vi "NanotecSMCPD.get axis status.vi"(0 "i ref in":refnum<vi>, 1 "axis":i32, 3 "ms timeout (10000)":i32=10000, 5 "error in (no error)":errorcluster) -> (14 "i ref out":refnum<vi>, 15 "status":T1=1 items=["motorEnabled"=1, "negativeLimitSwitchActive"=2, "positiveLimitSwitchActive"=4, "limitSwitchesEnabled"=8, "limitSwitchesAreNormallyClosed"=16, "moving"=32, "referenced"=64, "inPosition"=128, "reserved2"=256, "reserved3"=512, "reserved4"=1024, "reserved5"=2048, "error"=4096, "reserved6"=8192, "reserved7"=16384, "reserved8"=32768, "user defined1"=65536, "user defined2"=131072, "user defined3"=262144, "user defined4"=524288, "user defined5"=1048576, "user defined6"=2097152, "user defined7"=4194304, "user defined8"=8388608, "user defined9"=16777216, "user defined10"=33554432, "user defined11"=67108864, "user defined12"=134217728, "user defined13"=268435456, "user defined14"=536870912, "user defined15"=1073741824, "user defined16"=2147483648], 16 "motorOn":bool, 17 "timed out":bool, 19 "error out":errorcluster)   [LabVIEW 2014, in "NanotecSMCPD.lvlib"]
doc: "Gets the 32bit status byte of the specified axis."
uses:
  NanotecSMCPD.lvlib
  CSCore/CSApplicationBaseClasses/MotorBase/MotorBase.statusType.ctl
  CSCore/CSSystem/CoreDefs/CoreDefs.error_type.ctl
  CSCore/CSSystem/CoreDefs/CoreDefs.error_severity.ctl
  CSCore/CSApplicationBaseClasses/MotorBase/MotorBase.directionType.ctl
  CSCore/CSApplicationBaseClasses/MotorBase/MotorBase.serviceType.ctl
  CSlibraries/UtilityLib/UtilityLib.valueStatus.ctl
  CSCore/CSApplicationBaseClasses/DeviceBase/DeviceBase.lvlib
  CSCore/CSSystem/CoreLib/CoreLib.lvlib
  CSCore/CSApplicationBaseClasses/MotorBase/MotorBase.lvlib
  CSlibraries/UtilityLib/UtilityLib.lvlib
  CSinstr.lib/NanotecSMCPD/NanotecSMCPDDriver.lvlib
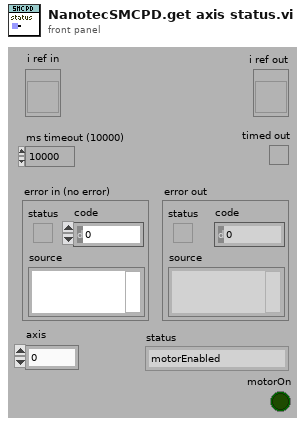
[diagram p1: front panel]
types:
  T1 = typedef "MotorBase.lvlib/MotorBase.statusType.ctl" = u32
  T2 = typedef "CoreDefs.error_severity.ctl" = enum16{"undefined", "information", "warning", "error", "fatal"}
  T3 = typedef "CoreDefs.error_type.ctl" = enum16{"no error", "can't load process", "can't unload process", "process does not exist", "can't install process", "can't remove process", "unknown function", "time out", "can't execute function", "duplicate queue name", "super not found", "caller queue invalid", "can't ping process", "unknown error", "VISA Error", "VISA timeout", "GPIB timeout", "GPIB error", "communication error", "data type mismatch", "can't read data from OPC server", "can't write data to OPC server", "OET error", "function not implemented", "process already exists", "invalid Shared Variable name", "error writing Shared Variable", "error reading Shared Variable", "invalid client name", "corrupt database", "unknown class", "call not authorized", "parameter out of range", "OET timeout: can't get data to modify", "invalid queue name", "requested operation incompatible with current state", "event undefined", "event disabled", "state undefined", "caller is not a friend", "EventBuilder: bad eventID", "EventBuilder: no DAQ devices", "a thread must not stop itself", "UNUSED ELEMENT4", "DiscArchiver: eventData incomplete", "DiscArchiver: eventData does not belong to run", "DiscArchiver: can't open file", "DiscArchiver: can't write to file", "DiscArchiver: available disc space low", "can't acquire semaphore", "error reading data from database", "notifier object is not existing", "can't register process", "can't unregister process", "illegal event type", "object disabled", "object already exists", "can't change state", "Instrument not found", "no connection to remote node", "invalid reference", "N/A", "UNUSED ELEMENT 1", "element not found", "illegal TCP/IP connection detected", "object does not exist", "invalid access ID", "unknown CS system", "invalid privilige", "unsupported data type", "unsupported server type", "IO server already exists", "Shared Variable already exists"}
  T4 = typedef "MotorBase.lvlib/MotorBase.serviceType.ctl" = enum16{"onOff", "startVelocity", "stopVelocity", "acceleration", "rangeMin", "rangeMax", "status", "position"}
  T5 = typedef "UtilityLib.lvlib/UtilityLib.valueStatus.ctl" = enum16{"no info available", "stand by/off", "on", "warning", "alarm/malfunction", "not implemented", "user action required", "important information", "system default", "control default", "indicator default", "button default"}
  T6 = typedef "MotorBase.lvlib/MotorBase.directionType.ctl" = enum16{"unknown", "update actual value", "update nominal value", "update both"}
  T7 = typedef "NanotecSMCPDDriver.lvlib/NanotecSMCPDDriver.status type.ctl" = cluster{"ready":bool, "homePosition":bool, "positionError":bool, "input1":bool, "controllerMode":enum16{"unknown", "position", "speed", "flagPosition", "clockDirection", "analog", "joystick", "unused"}, "unused":bool}
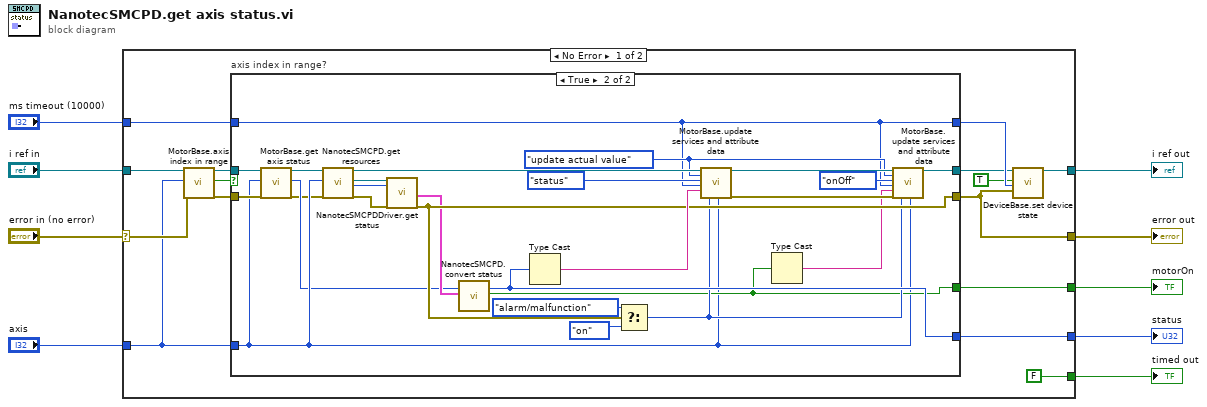
[diagram p0: block diagram]
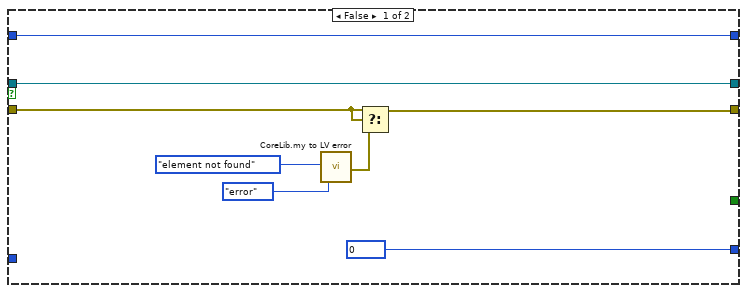
[diagram p2: hidden frame]
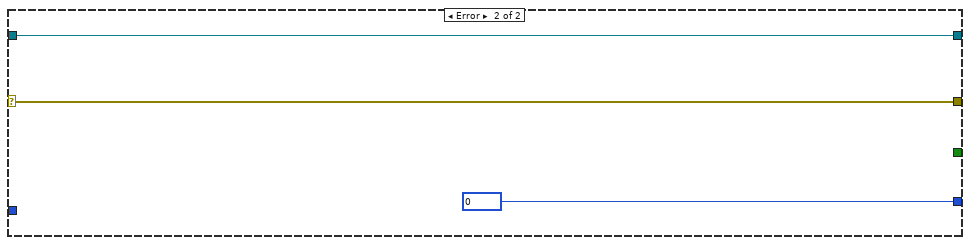
[diagram p3: hidden frame]
diagram:
  n1 = case shown="No Error" "error in (no error)" {
    selector: "error in (no error)" -> [w17 w60]
    tunnel: "ms timeout (10000)" -> [w14 _]
    tunnel: "i ref in" -> [w18 w61]
    tunnel: [w16 w60] -> w6
    tunnel: "axis" -> [w15 _]
    tunnel: [w13 w61] -> w4
    tunnel: [w12 w59] -> w3
    tunnel: [w11 _] -> w2
    tunnel: [FALSE _] -> w1
    frame No Error {
      n2 = call "MotorBase.axis index in range.vi"("i ref in"=w18, "axisIndex"=w15, "error in (no error)"=w17) -> ("i ref out"=w22:refnum<vi>, "in range"=w21:bool, "error out"=w23:errorcluster)  [unwired: 14 in]
      n3 = case "axis index in range?" shown="True" w21 {
        tunnel: [w32 w42] -> w20
        tunnel: [w29 w51] -> w16
        tunnel: w14 -> [w26 w45]
        tunnel: w15 -> [_ w37]
        tunnel: w22 -> [w32 w38]
        tunnel: w23 -> [w30 w39]
        tunnel: [w26 w45] -> w24
        tunnel: [w25 w50] -> w12
        tunnel: [_ w41] -> w11
        frame False {
          w25 = T1 0 items=["motorEnabled"=1, "negativeLimitSwitchActive"=2, "positiveLimitSwitchActive"=4, "limitSwitchesEnabled"=8, "limitSwitchesAreNormallyClosed"=16, "reseved1"=32, "referenced"=64, "inPosition"=128, "reserved2"=256, "reserved3"=512, "reserved4"=1024, "reserved5"=2048, "error"=4096, "reserved6"=8192, "reserved7"=16384, "reserved8"=32768, "user defined1"=65536, "user defined2"=131072, "user defined3"=262144, "user defined4"=524288, "user defined5"=1048576, "user defined6"=2097152, "user defined7"=4194304, "user defined8"=8388608, "user defined9"=16777216, "user defined10"=33554432, "user defined11"=67108864, "user defined12"=134217728, "user defined13"=268435456, "user defined14"=536870912, "user defined15"=1073741824, "user defined16"=2147483648] ("status")
          n4 = call "CoreLib.my to LV error.vi"("ErrorTypes"=CoreDefs.error_type."element not found", "severityLevel"=CoreDefs.error_severity."error") -> ("myErrorCluster"=w28:errorcluster)  [unwired: 16 in, 1 out]
          n5 = Select(t=w30, s=w30, f=w28) -> (s? t:f=w29:errorcluster)
        }
        frame True {
          w47 = MotorBase.directionType."update actual value" ("direction")
          n6 = call "MotorBase.get axis status.vi"("i ref in"=w38, "axisIndex"=w37, "error in (no error)"=w39) -> ("i ref out"=w34:refnum<vi>, "status"=w36:T1, "error out"=w35:errorcluster)  [unwired: 14 in]
          n7 = call "NanotecSMCPD.get resources.vi"("i ref in"=w34, "axisNumber"=w37, "error in (no error)"=w35) -> ("i ref out"=w54:refnum<vi>, "VISA resource"=w56:refnum<visa-resource-name>, "address"=w33:i32, "error out"=w55:errorcluster)  [unwired: 13 in]
          n8 = call "NanotecSMCPDDriver.get status.vi"("VISA resource name"=w56, "contollerID"=w33, "error in (no error)"=w55) -> ("actStatus"=w40:T7, "error out"=w51:errorcluster)  [unwired: 13 in, 2 out]
          n9 = call "NanotecSMCPD.convert status.vi"("status"=w36, "actStatus type"=w40) -> ("status out"=w50:T1, "motorOn"=w41:bool)  [unwired: 16 in]
          n10 = Type Cast(x=w50) -> (*(type *) &x=w58:string)  [unwired: 1 in]
          n11 = Select(t=UtilityLib.valueStatus."alarm/malfunction", s=w51, f=UtilityLib.valueStatus."on" ("quality")) -> (s? t:f=w43:T5)
          n12 = call "MotorBase.update services and attribute data.vi"("i ref in"=w54, "direction"=w47, "service"=MotorBase.serviceType."status", "ms timeout (10000)"=w45, "value"=w58, "quality"=w43, "axisNumber"=w37) -> ("i ref out"=w49:refnum<vi>, "error out"=w48:errorcluster)  [unwired: 10 in, 1 out]
          n13 = Type Cast(x=w41) -> (*(type *) &x=w44:string)  [unwired: 1 in]
          n14 = call "MotorBase.update services and attribute data.vi"("i ref in"=w49, "direction"=w47, "service"=MotorBase.serviceType."onOff", "ms timeout (10000)"=w45, "value"=w44, "error in (no error)"=w48, "quality"=w43, "axisNumber"=w37) -> ("i ref out"=w42:refnum<vi>)  [unwired: 9 in, 2 out]
        }
      }
      n15 = call "DeviceBase.set device state.vi"("i ref in"=w20, "implicit"=TRUE, "ms timeout (10000)"=w24, "device error"=w16) -> ("i ref out"=w13:refnum<vi>)  [unwired: 13 in, 2 out]
    }
    frame Error {
      w59 = T1 0 items=["motorEnabled"=1, "negativeLimitSwitchActive"=2, "positiveLimitSwitchActive"=4, "limitSwitchesEnabled"=8, "limitSwitchesAreNormallyClosed"=16, "reseved1"=32, "referenced"=64, "inPosition"=128, "reserved2"=256, "reserved3"=512, "reserved4"=1024, "reserved5"=2048, "error"=4096, "reserved6"=8192, "reserved7"=16384, "reserved8"=32768, "user defined1"=65536, "user defined2"=131072, "user defined3"=262144, "user defined4"=524288, "user defined5"=1048576, "user defined6"=2097152, "user defined7"=4194304, "user defined8"=8388608, "user defined9"=16777216, "user defined10"=33554432, "user defined11"=67108864, "user defined12"=134217728, "user defined13"=268435456, "user defined14"=536870912, "user defined15"=1073741824, "user defined16"=2147483648] ("status")
    }
  }
  "error out" <- w6
  "i ref out" <- w4
  "timed out" <- w1
  "status" <- w3
  "motorOn" <- w2
